vi "ReadMultiTof.vi"(8 "error in":errorcluster, 10 "VL6180 Resources":T1[](array[typedef]) {"I2C Slave Address" format="%02x"}, 11 "LINX Resource in":T2) -> (0 "error out":errorcluster, 1 "Distance Readings":u8[](array[numeric]), 2 "VL Configs":T1[](array[typedef]) {"I2C Slave Address" format="%02x"}, 3 "LINX Resource out":T2)   [LabVIEW 2014]
uses:
  Sensors/Time of Flight - VL6180/VL6180 Resource.ctl
  <vilib>/MakerHub/LINX/Private/Type Defs/LINX Ref.ctl
  <vilib>/MakerHub/LINX/Private/Type Defs/Platform.ctl
  <vilib>/MakerHub/LINX/Private/Type Defs/Interface.ctl
  <vilib>/MakerHub/LINX/Private/Device/Type Defs/LINX Device Config.ctl
  <vilib>/MakerHub/LINX/Private/Device/Type Defs/TCP Config.ctl
  <vilib>/MakerHub/LINX/Private/Device/Type Defs/Channels.ctl
  <vilib>/MakerHub/LINX/LMH-LINX.lvlib
  <vilib>/MakerHub/LINX/Private/Device/Device.lvlib
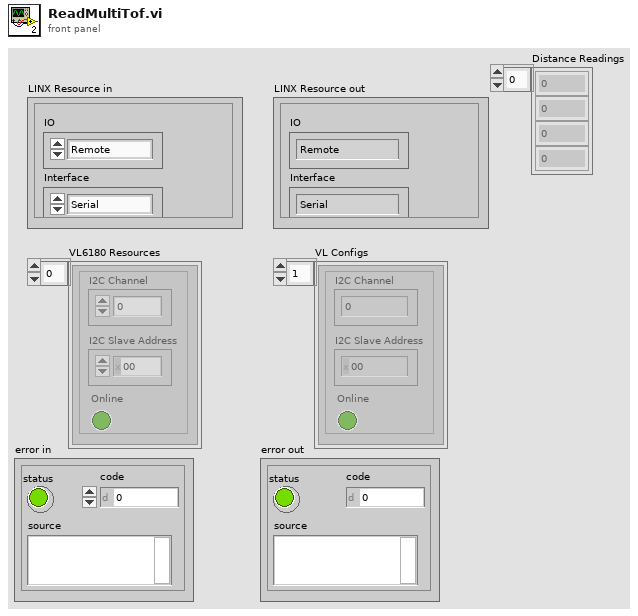
[diagram p1: front panel]
types:
  T1 = typedef "VL6180 Resource.ctl" = cluster{"I2C Channel":u8, "I2C Slave Address":u8, "Online":bool}
  T2 = typedef "LMH-LINX.lvlib/LINX Ref.ctl" = cluster{"IO":T3, "Interface":T4, "LINX Device Config":T5}
  T3 = typedef "LMH-LINX.lvlib/Platform.ctl" = enum16{"Remote", "Local"}
  T4 = typedef "LMH-LINX.lvlib/Interface.ctl" = enum16{"Serial", "TCP"}
  T5 = typedef "LMH-LINX.lvlib/Device.lvlib/LINX Device Config.ctl" = cluster{"Interface":T4, "COM Port":refnum<visa-resource-name>, "TCP Configuration":T6, "Device Family":u8, "Device ID":u8, "Device Name":string, "TCP Ref":refnum<k5>, "Channels":T7}
  T6 = typedef "LMH-LINX.lvlib/Device.lvlib/TCP Config.ctl" = cluster{"IP Address":string, "Port":u16}
  T7 = typedef "LMH-LINX.lvlib/Channels.ctl" = cluster{"DI":u8[], "DO":u8[], "AI":u8[], "AO":u8[], "PWM":u8[], "QE":u8[], "UART":u8[], "I2C 2":u8[], "SPI":u8[], "CAN":u8[], "Servo":u8[], "AI Ref (V)":dbl, "AI Resolution (Bits)":u8, "AO Ref (V)":dbl, "AO Resolution (Bits)":u8}
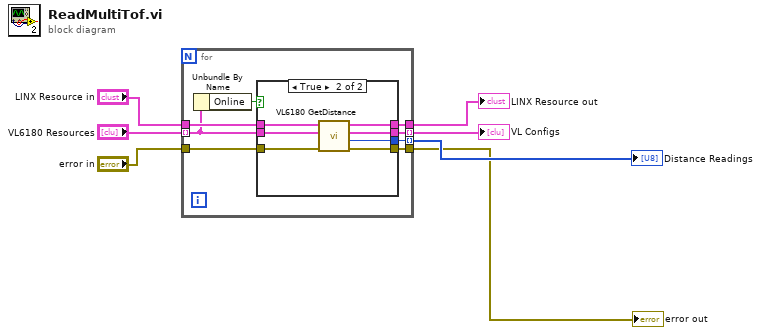
[diagram p0: block diagram]
diagram:
  n1 = for {
    tunnel: "VL6180 Resources" -> [w9] mode=indexing
    tunnel: "LINX Resource in" -> [w15]
    tunnel: "error in" -> [w12]
    tunnel: [w14] -> w6
    tunnel: [w13] -> w7 mode=indexing
    tunnel: [w11] -> w1
    tunnel: [w10] -> w2 mode=indexing
    n2 = Unbundle By Name(w9) -> ("Online"=w8:bool)
    n3 = case shown="True" w8 {
      tunnel: w15 -> [w18 w25]
      tunnel: w9 -> [w17 w24]
      tunnel: [w18 w23] -> w14
      tunnel: [w17 w22] -> w13
      tunnel: w12 -> [w16 w21]
      tunnel: [w16 w20] -> w11
      tunnel: [_ w19] -> w10
      frame False {
      }
      frame True {
        n4 = call "VL6180 GetDistance.vi"("error in (no error)"=w21, "VL6180 Resource in"=w24, "LINX Resource"=w25) -> ("error out"=w20:errorcluster, "Distance (mm)"=w19:u8, "VL6180 Resource out"=w22:T1, "LINX Resource"=w23:T2)  [unwired: 4 in, 1 out]
      }
    }
  }
  "error out" <- w1
  "VL Configs" <- w7
  "LINX Resource out" <- w6
  "Distance Readings" <- w2
